vi "CAN TPCANHandle-Channel-from-Enum_eX.vi"(11 "TPCANHandle-Channel":T1) -> (3 "Channel":u16 format="%x")   [LabVIEW 2020, in "PCANBasic_eX.lvlib"]
uses:
  PCANBasic_eX.lvlib
  CTLs/TPCANHandle-Channel_eX.ctl
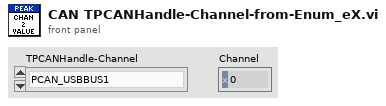
[diagram p1: front panel]
types:
  T1 = typedef "PCANBasic_eX.lvlib/TPCANHandle-Channel_eX.ctl" = enum16{"PCAN_USBBUS1", "PCAN_USBBUS2"}
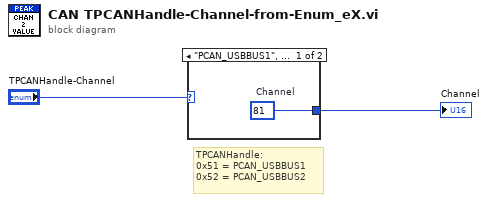
[diagram p0: block diagram]
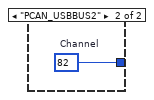
[diagram p2: hidden frame]
diagram:
  # "TPCANHandle:\n0x51 = PCAN_USBBUS1\n0x52 = PCAN_USBBUS2"
  n1 = case shown="\"PCAN_USBBUS1\", Default" "TPCANHandle-Channel" {
    tunnel: [w3 w4] -> w1
    frame "PCAN_USBBUS1", Default {
      w3 = u16 81  # Channel
    }
    frame "PCAN_USBBUS2" {
      w4 = u16 82  # Channel
    }
  }
  "Channel" <- w1
